vi "Z Aux Write U File.vi"(8 "error in (no error)":errorcluster caption="错误输入（无错误）", 9 "inum":i32, 10 "pVarlist":sgl, 11 "sFilename":string) -> (0 "error out":errorcluster caption="错误输出", 2 "pVarlist out":sgl, 3 "function return":i32)   [LabVIEW 2015, in "zauxdll.lvlib"]
doc: "int32 __stdcall ZAux_WriteUFile(const char *sFilename, float *pVarlist, int inum);"
uses:
  zauxdll.lvlib
  zauxdll.dll
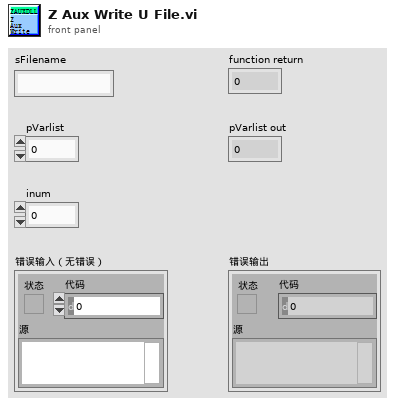
[diagram p1: front panel]
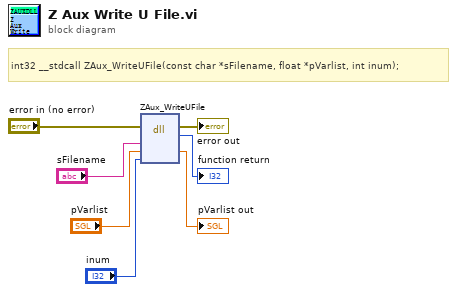
[diagram p0: block diagram]
diagram:
  # "int32 __stdcall ZAux_WriteUFile(const char *sFilename, float *pVarlist, int inum);"
  n1 = dll-call lib="C:/Users/VIC/Desktop/GOGORO_Oringnal - Panasonic/system/LLB/zmotion/zaux/zauxdll.*" fn="ZAux_WriteUFile"(error in="error in (no error)", "sFilename"="sFilename", "pVarlist"="pVarlist", "inum"="inum") -> (error out=→"error out":errorcluster, →"function return":i32, "pVarlist"=→"pVarlist out":sgl)  [unwired: 4 in, 1 out]
